vi "Initialize Steering Frame.vi"(8 "error in (no error)":errorcluster) -> (0 "error out":errorcluster, 3 "steering frame":refnum<data-value>)   [LabVIEW 2017, in "NI_Robotics_Configure Steering Frame.lvlib"]
uses:
  <vilib>/robotics/Dialog/Configure Steering Frame/NI_Robotics_Configure Steering Frame.lvlib
  <vilib>/robotics/Steering/Steering Frame/NI_Robotics_Steering Frame.lvclass
  <vilib>/robotics/Steering/Wheel/Wheel Parameters.ctl
  <vilib>/robotics/Steering/Wheel/Rotation Direction.ctl
  <vilib>/robotics/Steering/Fixed Wheel/NI_Robotics_Fixed Wheel.lvclass
  c:/Program Files (x86)/National Instruments/LabVIEW 2017/vi.lib/robotics/Steering/Wheel/NI_Robotics_Wheel.lvclass
  <vilib>/robotics/Steering/Steering Frame/Create User Defined Steering Frame.vi
  <vilib>/robotics/Steering/Fixed Wheel/Create Fixed Wheel.vi
  <vilib>/robotics/Steering/Wheel/NI_Robotics_Wheel.lvclass
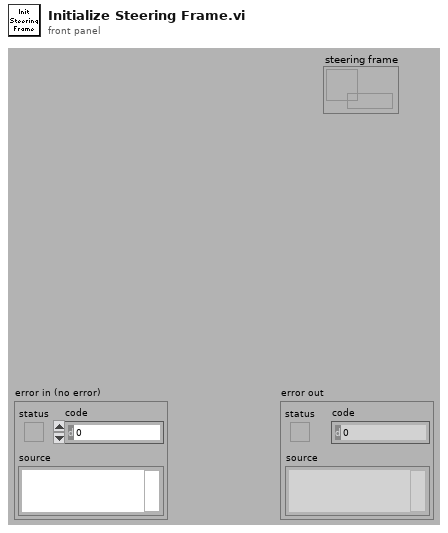
[diagram p1: front panel]
types:
  T1 = typedef "NI_Robotics_Wheel.lvclass/Wheel Parameters.ctl" = cluster{"wheel radius":dbl, "gear ratio":dbl, "forward rotation direction":T2}
  T2 = typedef "NI_Robotics_Wheel.lvclass/Rotation Direction.ctl" = u16
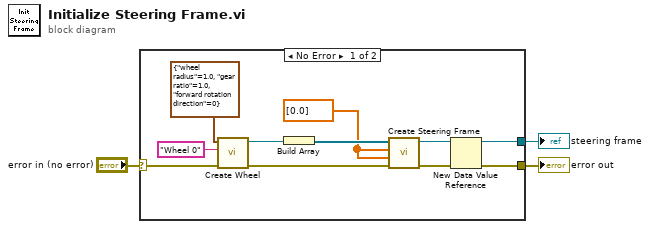
[diagram p0: block diagram]
diagram:
  n1 = case shown="No Error" "error in (no error)" {
    selector: "error in (no error)" -> [w14 w15]
    tunnel: [w7 w15] -> w2
    tunnel: [w6 _] -> w1
    frame No Error {
      w5 = dbl[] [0.0] ("wheel x positions")
      n2 = call-poly <vilib>:"Create Wheel.vi"("error in (no error)"=w14, "wheel name"="Wheel 0", "wheel parameters"=T1 {"wheel radius"=1.0, "gear ratio"=1.0, "forward rotation direction"=0}) -> ("error out"=w10:errorcluster, "fixed wheel out"=w12:refnum<class "NI_Robotics_Fixed Wheel.lvclass">)  [unwired: 7 in]
      n3 = Build Array(w12) -> (w13:refnum<class "NI_Robotics_Fixed Wheel.lvclass">[])
      n4 = call-poly <vilib>:"Create Steering Frame.vi"("error in (no error)"=w10, "wheel y positions"=w5, "wheel x positions"=w5, "wheels"=w13) -> ("error out"=w8:errorcluster, "steering frame out"=w9:refnum<class "NI_Robotics_Steering Frame.lvclass">)  [unwired: 6 in]
      n5 = New Data Value Reference(data value=w9, error in=w8) -> (data value reference=w6:refnum<data-value>, error out=w7:errorcluster)
    }
    frame Error {
    }
  }
  "error out" <- w2
  "steering frame" <- w1
